vi "Configure Buffering.vi"(8 "error in (no error)":errorcluster, 9 "Enable Buffering (Enable)":bool, 11 "VISA resource name":refnum<visa-resource-name>) -> (0 "error out":errorcluster, 2 "Confirmation Response":string, 3 "VISA resource name out":refnum<visa-resource-name>)   [LabVIEW 2024, in "Micron Optics sm130.lvlib"]
doc: "Configures the streaming mode for the instrument. During streaming mode, the instrument will generate the GET_DATA command internally. In order to extract data, only a read is required. The instrument will not respond to messages so that there is no desynchronization of the data that is being passed.\n\nIf a Read VI besides the Read Streaming Data is run, there will be an error. Therefore, disable streaming mode before using the other read vi's."
uses:
  Micron Optics sm130.lvlib
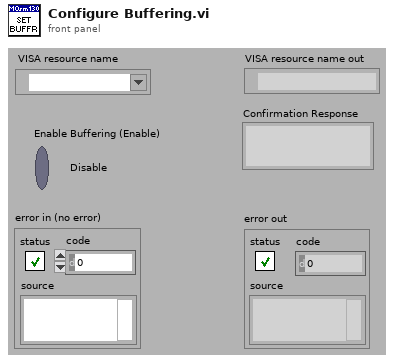
[diagram p1: front panel]
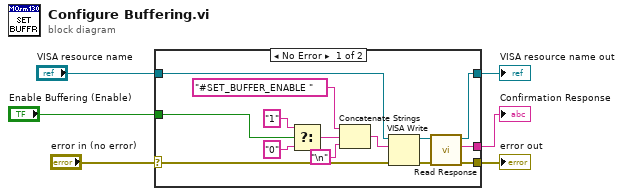
[diagram p0: block diagram]
diagram:
  n1 = case shown="No Error" "error in (no error)" {
    selector: "error in (no error)" -> [w8 w22]
    tunnel: "VISA resource name" -> [w20 w21]
    tunnel: [w19 w21] -> w5
    tunnel: [w18 w22] -> w4
    tunnel: "Enable Buffering (Enable)" -> [w17 _]
    tunnel: [w9 _] -> w2
    frame No Error {
      n2 = Select(t="1" ("write buffer"), s=w17, f="0" ("write buffer")) -> (s? t:f=w11:string)
      n3 = Concatenate Strings("#SET_BUFFER_ENABLE " ("write buffer"), w11, "\n") -> (w10:string)
      n4 = VISA Write(VISA resource name=w20, write buffer=w10, error in (no error)=w8) -> (VISA resource name out=w16:refnum<visa-resource-name>, error out=w15:errorcluster)  [unwired: 1 out]
      n5 = call "Read Response.vi"("error in (no error)"=w15, "VISA resource name"=w16) -> ("error out"=w18:errorcluster, "Confirmation Response"=w9:string, "VISA resource name out"=w19:refnum<visa-resource-name>)  [unwired: 7 in]
    }
    frame Error {
    }
  }
  "VISA resource name out" <- w5
  "error out" <- w4
  "Confirmation Response" <- w2
